vi "Get StateChange N Chains.vi"(8 "error in (no error)":errorcluster, 11 "niDTS WLAN DUT in":refnum<class "niDTS WLAN Dut.lvclass">) -> (0 "error out":errorcluster, 2 "Changed":bool, 3 "niDTS WLAN DUT out":refnum<class "niDTS WLAN Dut.lvclass">)   [LabVIEW 2015, in "niDTS WLAN.lvlib" / "niDTS WLAN Dut.lvclass"]
uses:
  niDTS WLAN Dut.lvclass
  niDTS WLAN Dut Data/niDTS WLAN Dut Data.lvclass
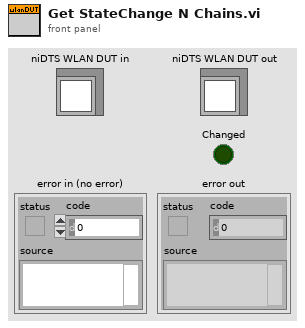
[diagram p1: front panel]
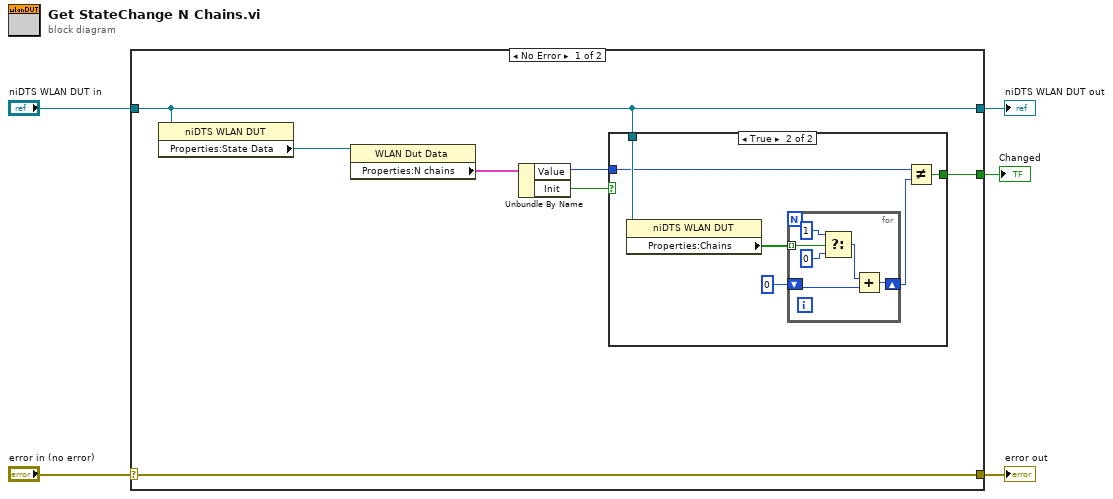
[diagram p0: block diagram]
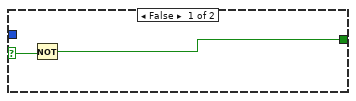
[diagram p2: hidden frame]
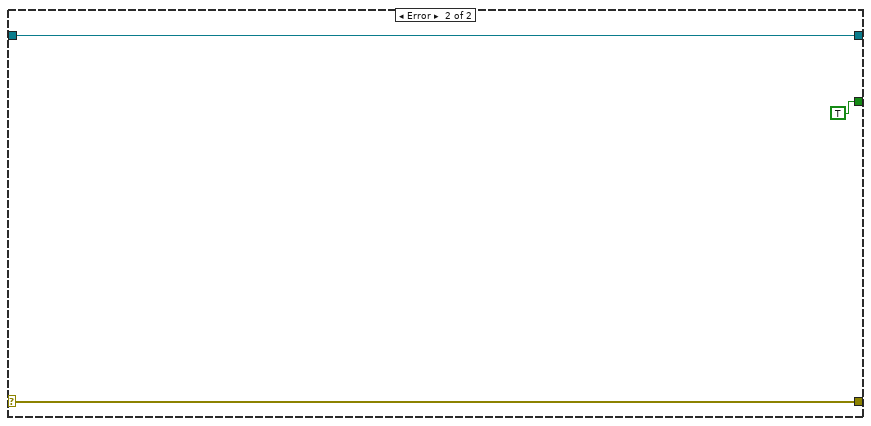
[diagram p3: hidden frame]
diagram:
  n1 = case shown="No Error" "error in (no error)" {
    selector: "error in (no error)" -> [w12 w29]
    tunnel: [w12 w29] -> w4
    tunnel: [w6 w28] -> w1
    tunnel: "niDTS WLAN DUT in" -> [w6 w28]
    tunnel: [w8 TRUE] -> w2
    frame No Error {
      n2 = property class="niDTS WLAN DUT"(reference=w6) -> ("Properties:State Data"=w11:refnum<class "niDTS WLAN Dut Data.lvclass">)  [unwired: 1 in, 2 out]
      n3 = property class="WLAN Dut Data"(reference=w11) -> ("Properties:N chains"=w10:cluster{"Value":i32, "Init":bool})  [unwired: 1 in, 2 out]
      n4 = Unbundle By Name(w10) -> ("Value"=w7:i32, "Init"=w9:bool)
      n5 = case shown="True" w9 {
        selector: w9 -> [w14 _]
        tunnel: [w13 w18] -> w8
        tunnel: w7 -> [_ w19]
        tunnel: w6 -> [_ w20]
        frame False {
          n6 = Not(x=w14) -> (.not. x?=w13:bool)
        }
        frame True {
          n7 = property class="niDTS WLAN DUT"(reference=w20) -> ("Properties:Chains"=w17:bool[])  [unwired: 1 in, 2 out]
          n8 = for {
            tunnel: w17 -> [w26] mode=indexing
            shift-right: [w23] -> w15
            shift-left: 0 ("Value") -> [w22]
            n9 = Select(t=1 ("Value"), s=w26, f=0 ("Value")) -> (s? t:f=w21:i32)
            n10 = Add(x=w21, y=w22) -> (x+y=w23:i32)
          }
          n11 = Not Equal?(x=w19, y=w15) -> (x != y?=w18:bool)
        }
      }
    }
    frame Error {
    }
  }
  "error out" <- w4
  "niDTS WLAN DUT out" <- w1
  "Changed" <- w2
